vi "Acquisition Message Loop.vi"(8 "error in (no error)":errorcluster, 9 "Data Queue":refnum<queue>, 10 "Data Notifier":refnum<notifier>, 11 "Message Queues":T1) -> (0 "error out":errorcluster)   [LabVIEW 2023, in "Acquisition.lvlib"]
doc: "Message loop for handling messages pertaining to the acquisition of data from the hardware."
uses:
  Acquisition.lvlib
  support/Message Queue/All Message Queues.ctl
  support/Message Queue/Message Cluster.ctl
  Hardware Configuration.ctl
  Signal Type.ctl
  Acquisition State.ctl
  support/Message Queue/Enqueue Message (Single).vi
  <vilib>/Utility/error.llb/Error Cluster From Error Code.vi
  <vilib>/ErrorRing/Error Ring.xnode
  support/Message Queue/Message Queue.lvlib
panel:
  out "millisecond timer value":u32
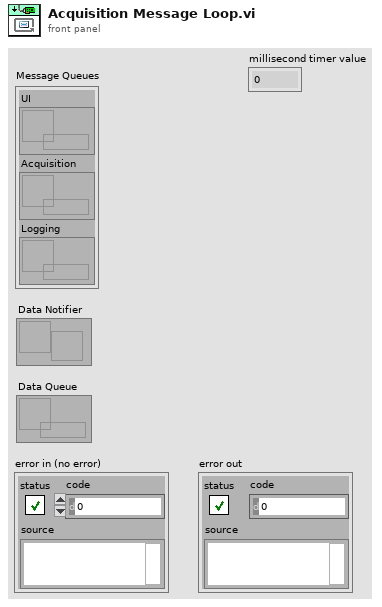
[diagram p1: front panel]
types:
  T1 = typedef "Message Queue.lvlib/All Message Queues.ctl" = cluster{"UI":refnum<queue>, "Acquisition":refnum<queue>, "Logging":refnum<queue>}
  T2 = typedef "Acquisition.lvlib/Hardware Configuration.ctl" = cluster{"AIDAQ":refnum<k21>, "Signal Type":T3, "DODAQ":refnum<k21>}
  T3 = typedef "Acquisition.lvlib/Signal Type.ctl" = enum16{"cDAQ RTD", "myDAQ Temp", "Sine Wave", "Square with Noise"}
  T4 = typedef "Acquisition.lvlib/Acquisition State.ctl" = enum16{"Idle", "Acquiring"}
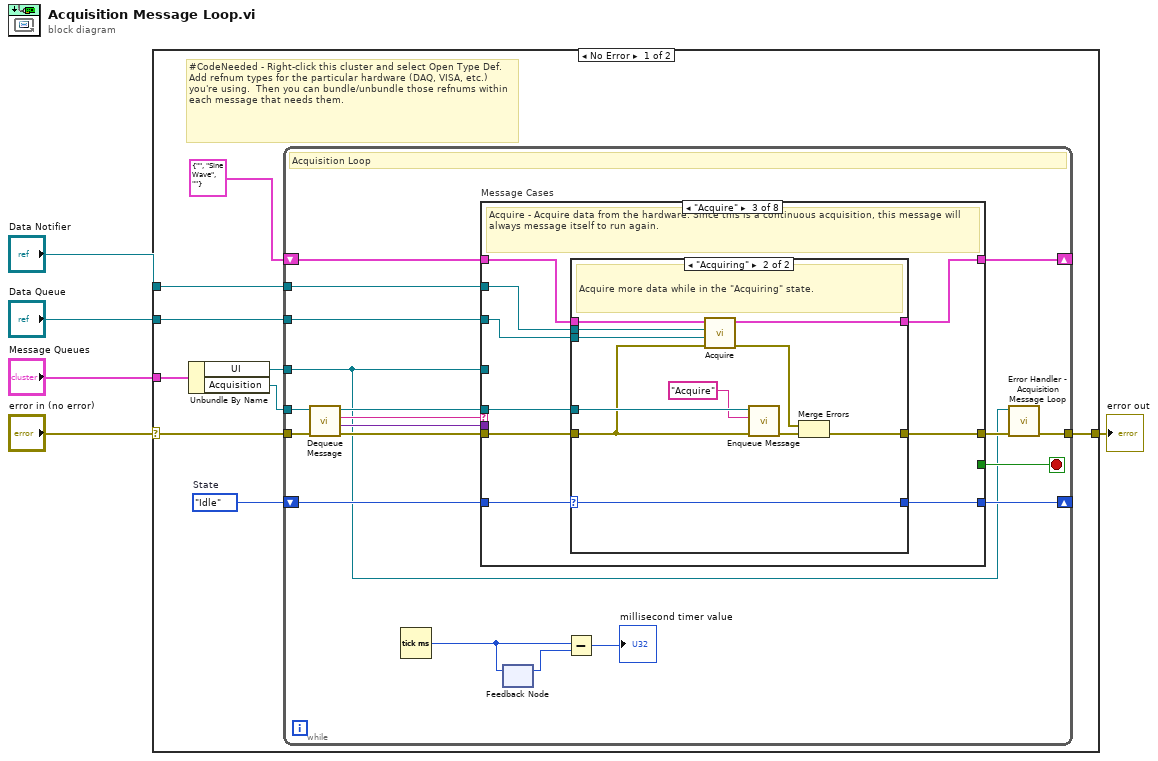
[diagram p0: block diagram]
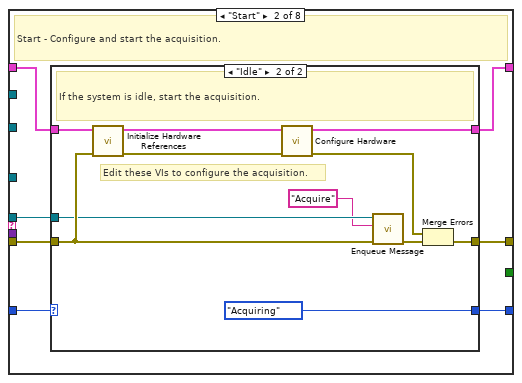
[diagram p3: hidden frame]
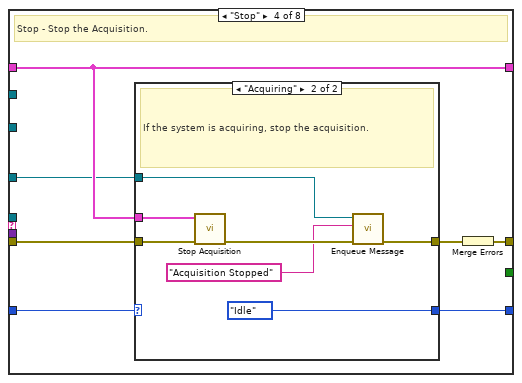
[diagram p6: hidden frame]
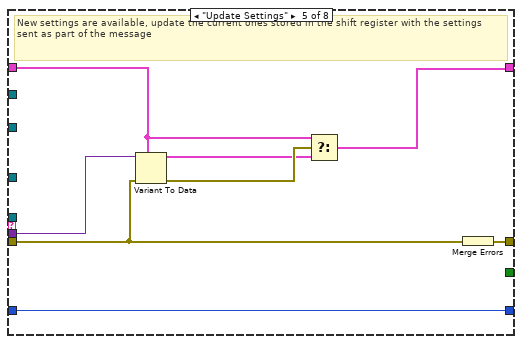
[diagram p8: hidden frame]
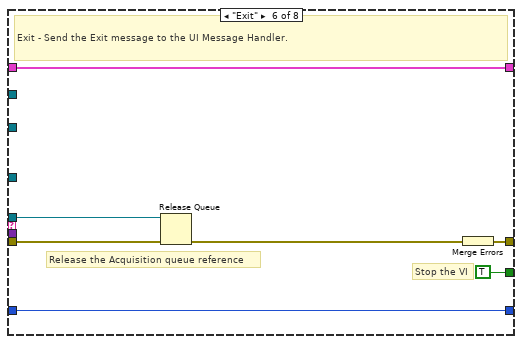
[diagram p9: hidden frame]
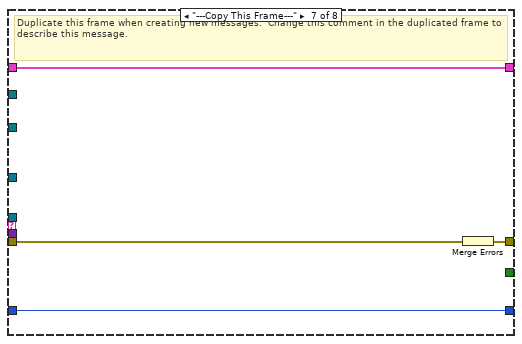
[diagram p10: hidden frame]
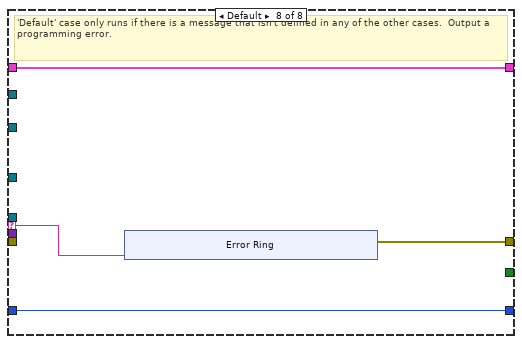
[diagram p11: hidden frame]
diagram:
  n1 = case shown="No Error" "error in (no error)" {
    selector: "error in (no error)" -> [w10 w127]
    tunnel: "Message Queues" -> [w14 _]
    tunnel: [w12 w127] -> w4
    tunnel: "Data Notifier" -> [w8 _]
    tunnel: "Data Queue" -> [w7 _]
    frame No Error {
      w6 = Acquisition_State."Idle"  # State
      # "#CodeNeeded - Right-click this cluster and select Open Type Def.  Add refnum types for the particular hardware (DAQ, VISA, etc.) you're using.  Then you can bundle/unbundle those refnums within each message that needs them."
      n2 = Unbundle By Name(w14) -> ("UI"=w9:refnum<queue>, "Acquisition"=w13:refnum<queue>)
      n3 = while {
        tunnel: w13 -> [w26]
        shift-right: [w32] -> _
        shift-left: T2 {"AIDAQ"="", "Signal Type"=enum."Sine Wave", "DODAQ"=""} ("Data Cluster") -> [w33]
        tunnel: w9 -> [w18]
        tunnel: w8 -> [w25]
        tunnel: w7 -> [w24]
        shift-right: [w22] -> _
        shift-left: w6 -> [w23]
        tunnel: w10 -> [w30]
        tunnel: [w21] -> w12
        stop <- w31 stop-if-true
        # "Acquisition Loop"
        n4 = call "Dequeue Message.vi"("error in (no error)"=w30, "Message Queue"=w26) -> ("error out"=w29:errorcluster, "Message Data"=w27:variant, "Message"=w28:string, "dup Message Queue"=w19:refnum<queue>)  [unwired: 6 in]
        n5 = Tick Count (ms)() -> (millisecond timer value=w15:u32)
        n6 = case "Message Cases" shown="\"Acquire\"" w28 {
          selector: w28 -> [_ _ _ _ _ _ _ w116]
          tunnel: w19 -> [_ w40 w65 _ _ w106 _ _]
          tunnel: w29 -> [w36 w41 w64 w86 w98 w108 w115 _]
          tunnel: [w36 w43 w66 w87 w104 w110 w113 w117] -> w20
          tunnel: w33 -> [w35 w42 w62 w84 w100 w109 w114 w119]
          tunnel: [w35 w39 w63 w84 w99 w109 w114 w119] -> w32
          tunnel: [_ _ _ _ _ TRUE _ _] -> w31
          tunnel: w27 -> [_ _ _ _ w103 _ _ _]
          tunnel: w18 -> [_ _ _ w81 _ _ _ _]
          tunnel: w25 -> [_ _ w61 _ _ _ _ _]
          tunnel: w24 -> [_ _ w60 _ _ _ _ _]
          tunnel: w23 -> [w34 w37 w58 w83 w97 w105 w112 w118]
          tunnel: [w34 w38 w59 w82 w97 w105 w112 w118] -> w22
          frame "Initialize" {
            # "Initialize  - Initialize is currently a no-op.  The hardware initialization takes place in the 'Start' message."
          }
          frame "Start" {
            # "Start - Configure and start the acquisition."
            n7 = case shown="\"Idle\"" w37 {
              selector: w37 -> [w44 _]
              tunnel: [w45 w57] -> w43
              tunnel: w42 -> [w46 w56]
              tunnel: w41 -> [w45 w55]
              tunnel: w40 -> [_ w53]
              tunnel: [w46 w49] -> w39
              tunnel: [w44 Acquisition_State."Acquiring" ("Acquisition State")] -> w38
              frame "Acquiring" {
                # "The system is already acquiring. Ignore the \"Start\" message."
              }
              frame "Idle" {
                # "Edit these VIs to configure the acquisition."
                # "If the system is idle, start the acquisition."
                n8 = call "Initialize Hardware References.vi"("error in (no error)"=w55, "Hardware Resources in"=w56) -> ("error out"=w52:errorcluster, "Hardware Resources out"=w50:T2)  [unwired: 8 in]
                n9 = call "Configure Hardware.vi"("error in (no error)"=w52, "Hardware Resources in"=w50) -> ("error out"=w51:errorcluster, "Hardware Resources out"=w49:T2)  [unwired: 8 in]
                n10 = call-poly "Enqueue Message.vi"("error in (no error)"=w55, "Message"="Acquire", "Message Queue"=w53) -> ("error out"=w54:errorcluster)  [unwired: 7 in, 1 out]
                n11 = Merge Errors(w51, w54) -> (w57:errorcluster)
              }
            }
          }
          frame "Acquire" {
            # "Acquire - Acquire data from the hardware. Since this is a continuous acquisition, this message will always message itself to run again."
            n12 = case shown="\"Acquiring\"" w58 {
              selector: w58 -> [w67 w71]
              tunnel: [w68 w80] -> w66
              tunnel: w65 -> [_ w78]
              tunnel: w64 -> [w68 w70]
              tunnel: [w69 w76] -> w63
              tunnel: w62 -> [w69 w75]
              tunnel: w61 -> [_ w73]
              tunnel: w60 -> [_ w72]
              tunnel: [w67 w71] -> w59
              frame "Idle" {
                # "Ignore \"Acquire\" messages when the acquisition is idle."
              }
              frame "Acquiring" {
                # "Acquire more data while in the \"Acquiring\" state."
                n13 = call "Acquire.vi"("error in (no error)"=w70, "Data Queue"=w72, "Data Notifier"=w73, "Hardware Resources in"=w75) -> ("error out"=w77:errorcluster, "Hardware Resources out"=w76:T2)  [unwired: 6 in]
                n14 = call-poly "Enqueue Message.vi"("error in (no error)"=w70, "Message"="Acquire", "Message Queue"=w78) -> ("error out"=w79:errorcluster)  [unwired: 7 in, 1 out]
                n15 = Merge Errors(w77, w79) -> (w80:errorcluster)
              }
            }
          }
          frame "Stop" {
            # "Stop - Stop the Acquisition."
            n16 = case shown="\"Acquiring\"" w83 {
              selector: w83 -> [w88 _]
              tunnel: w86 -> [w89 w96]
              tunnel: [w89 w92] -> w85
              tunnel: w84 -> [_ w94]
              tunnel: [w88 Acquisition_State."Idle" ("State")] -> w82
              tunnel: w81 -> [_ w91]
              frame "Idle" {
                # "The system is already idle. Ignore the \"Stop\" message."
              }
              frame "Acquiring" {
                # "If the system is acquiring, stop the acquisition."
                n17 = call "Stop Acquisition.vi"("error in (no error)"=w96, "Hardware Resources in"=w94) -> ("error out"=w95:errorcluster)  [unwired: 9 in]
                n18 = call-poly "Enqueue Message.vi"("error in (no error)"=w95, "Message"="Acquisition Stopped", "Message Queue"=w91) -> ("error out"=w92:errorcluster)  [unwired: 7 in, 1 out]
              }
            }
            n19 = Merge Errors(w85) -> (w87:errorcluster)
          }
          frame "Update Settings" {
            # "New settings are available, update the current ones stored in the shift register with the settings sent as part of the message"
            n20 = Variant To Data(error in=w98, type=w100, Variant=w103) -> (data=w101:T2, error out=w102:errorcluster)
            n21 = Select(t=w100, s=w102, f=w101) -> (s? t:f=w99:T2)
            n22 = Merge Errors(w98) -> (w104:errorcluster)
          }
          frame "Exit" {
            # "Release the Acquisition queue reference"
            # "Stop the VI"
            # "Exit - Send the Exit message to the UI Message Handler."
            n23 = Release Queue(queue=w106, error in (no error)=w108) -> (error out=w107:errorcluster)  [unwired: 1 in, 2 out]
            n24 = Merge Errors(w107) -> (w110:errorcluster)
          }
          frame "---Copy This Frame---" {
            # "Duplicate this frame when creating new messages.  Change this comment in the duplicated frame to describe this message."
            n25 = Merge Errors(w115) -> (w113:errorcluster)
          }
          frame Default {
            # "'Default' case only runs if there is a message that isn't defined in any of the other cases.  Output a programming error."
            n26 = xnode "Error Ring"("parameter 0"=w116) -> ("error out"=w117:errorcluster)
          }
        }
        n27 = feedback-in #1(w15) -> ()
        n28 = feedback #1() -> (w16:u32)  [unwired: 1 in]
        n29 = Subtract(x=w15, y=w16) -> (x-y=→"millisecond timer value":u32)
        n30 = call "Error Handler - Acquisition Message Loop.vi"("error in (no error)"=w20, "Message Queue"=w18) -> ("dup error in"=w21:errorcluster)  [unwired: 8 in, 1 out]
      }
    }
    frame Error {
    }
  }
  "error out" <- w4
